vi "ImageBrowser.vi"() -> ()   [LabVIEW 2016]
doc: "This example shows how to set up an image browser. An image browser is a concise representation of the images in your database represented as thumbnails on a page. You can use the Browser VIs in NI Vision to configure a browser, configure the selection of one or many images, add new images and remove images to and from a browser, replace an image, and get or set the selection status of an image."
uses:
  <vilib>/vision/NI_Vision_Development_Module.lvlib
panel:
  out "Images":T1(plugin-control)
  in  "Stop":bool
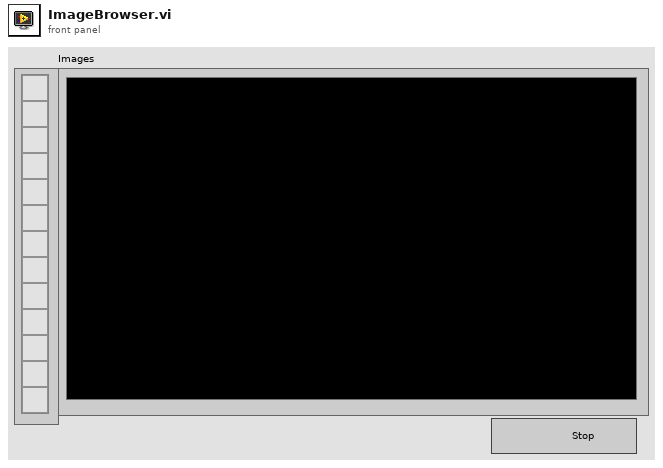
[diagram p1: front panel]
types:
  T1 = typedef "IMAQ Image.ctl" = refnum<image>
  T2 = cluster{"Browser\nSize":cluster{"X":i32, "Y":i32}, "Images per Line":i32, "Background Color":u32, "Frame Size":i32, "Frame Style":u16}
  T3 = typedef "Image Type" = u32
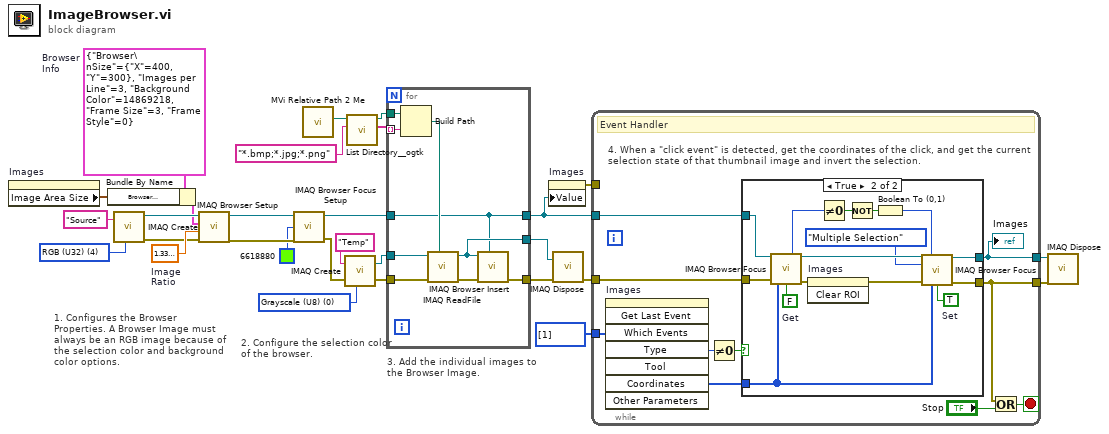
[diagram p0: block diagram]
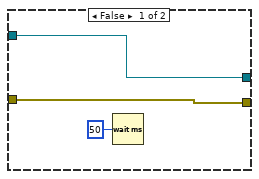
[diagram p2: hidden frame]
diagram:
  w18 = i32[] [1] items=["No Event"=0, "Click Event"=1, "Draw Event"=2, "Size Event"=4, "Scroll Event"=5, "Double Click Event"=8] ("Which Events")
  w29 = sgl 1.33  # Image  Ratio
  w8 = T2 {"Browser\nSize"={"X"=400, "Y"=300}, "Images per Line"=3, "Background Color"=14869218, "Frame Size"=3, "Frame Style"=0}  # Browser Info
  w22 = T3 0 items=["Grayscale (U8)", "Grayscale (I16)", "Grayscale (SGL)", "Complex (CSG)", "RGB (U32)", "HSL (U32)", "RGB (U64)", "Grayscale (U16)"] ("Image Type")
  w24 = T3 4 items=["Grayscale (U8)", "Grayscale (I16)", "Grayscale (SGL)", "Complex (CSG)", "RGB (U32)", "HSL (U32)", "RGB (U64)", "Grayscale (U16)"] ("Image Type")
  # "3. Add the individual images to the Browser Image."
  # "2. Configure the selection color of the browser."
  # "1. Configures the Browser Properties. A Browser Image must always be an RGB image because of the selection color and background color options."
  n1 = property on="Images" class="ImageControl"() -> ("Image Area Size"=w7:cluster{"Width":u32, "Height":u32})  [unwired: 2 in, 2 out]
  n2 = Bundle By Name(cluster=w8, "Browser\nSize"=w7) -> (w6:T2)
  n3 = call "IMAQ Create"("Image Name"="Source", "Image Type"=w24) -> ("New Image"=w26:T1, "error out"=w25:errorcluster)  [unwired: 3 in]
  n4 = call "IMAQ Browser Setup"("error in (no error)"=w25, "Image Ratio"=w29, "Browser Info"=w6, "Image In"=w26) -> ("error out"=w12:errorcluster, "Image Browser Out"=w13:T1)  [unwired: 2 out]
  n5 = call "IMAQ Browser Focus Setup"("error in (no error)"=w12, "Focus Color"=u32 6618880, "Image Browser In"=w13) -> ("error out"=w10:errorcluster, "Image Browser Out"=w11:T1)  [unwired: 1 in]
  n6 = call "MVi Relative Path 2 Me.vi"() -> ("MyDir"=w1:path)  [unwired: 6 in, 1 out]
  n7 = call "IMAQ Create"("Image Name"="Temp", "Image Type"=w22, "error in (no error)"=w10) -> ("New Image"=w15:T1, "error out"=w28:errorcluster)  [unwired: 2 in]
  n8 = call "List Directory__ogtk.vi"("pattern"="*.bmp;*.jpg;*.png", "directory path"=w1) -> ("file names"=w2:string[], "dup directory path"=w4:path)  [unwired: 2 in, 2 out]
  n9 = for {
    tunnel: w11 -> [w30]
    tunnel: w4 -> [w38]
    tunnel: w2 -> [w35] mode=indexing
    tunnel: w28 -> [w34]
    tunnel: [w33] -> w27
    tunnel: [w30] -> w19
    tunnel: w15 -> [w32]
    tunnel: [w31] -> w14
    n10 = Build Path(base path=w38, name or relative path=w35) -> (appended path=w37:path)
    n11 = call "IMAQ ReadFile"("File Path"=w37, "error in (no error)"=w34, "Image"=w32) -> ("error out"=w36:errorcluster, "Image Out"=w31:T1)  [unwired: 4 in, 3 out]
    n12 = call "IMAQ Browser Insert"("Image Browser In"=w30, "error in (no error)"=w36, "Image to Add"=w31) -> ("error out"=w33:errorcluster)  [unwired: 4 in, 4 out]
  }
  n13 = property on="Images" class="ImageControl"("Value"=w19) -> (error out=w5:errorcluster)  [unwired: 2 in, 1 out]
  n14 = call "IMAQ Dispose"("Image"=w14, "error in (no error)"=w27) -> ("error out"=w20:errorcluster)  [unwired: 4 in]
  n15 = while {
    tunnel: w19 -> [w48]
    tunnel: w20 -> [w45]
    tunnel: w18 -> [w46]
    tunnel: [w43] -> w17
    tunnel: [w40] -> w16
    tunnel: w5 -> [_]
    stop <- w41 stop-if-true
    # "4. When a \"click event\" is detected, get the coordinates of the click, and get the current selection state of that thumbnail image and invert the selection."
    # "Event Handler"
    n16 = invoke on="Images" class="ImageControl" method="Get Last Event"("Which Events"=w46) -> ("Type"=w39:i32, "Coordinates"=w47:i32[])  [unwired: 7 in, 6 out]
    n17 = Not Equal To 0?(x=w39) -> (x != 0?=w44:bool)
    n18 = case shown="True" w44 {
      tunnel: w48 -> [w50 w66]
      tunnel: w47 -> [_ w57]
      tunnel: w45 -> [w51 w56]
      tunnel: [w51 w55] -> w43
      tunnel: [w50 w54] -> w40
      frame False {
        n19 = Wait (ms)(milliseconds to wait=u32 50) -> ()  [unwired: 1 out]
      }
      frame True {
        w64 = TRUE  # Set
        w65 = FALSE  # Get
        n20 = call "IMAQ Browser Focus"("Image Browser In"=w66, "error in (no error)"=w56, "Pixel Position"=w57, "Get/Set (Set)"=w65) -> ("State Out"=w61:enum16{"Not selected", "Selected"}, "Image Browser Out"=w63:T1, "error out"=w53:errorcluster)  [unwired: 6 in, 3 out]
        n21 = invoke on="Images" class="ImageControl" method="Clear ROI"(error in=w53) -> (error out=w52:errorcluster)  [unwired: 2 in, 2 out]
        n22 = Not Equal To 0?(x=w61) -> (x != 0?=w59:bool)
        n23 = Not(x=w59) -> (.not. x?=w58:bool)
        n24 = Boolean To (0,1)(Boolean=w58) -> (0, 1=w60:i16)
        n25 = call "IMAQ Browser Focus"("Image Browser In"=w63, "State In"=w60, "Selection Mode"=enum16{"Single Selection", "Multiple Selection"}."Multiple Selection", "error in (no error)"=w52, "Pixel Position"=w57, "Get/Set (Set)"=w64) -> ("Image Browser Out"=w54:T1, "error out"=w55:errorcluster)  [unwired: 4 in, 4 out]
      }
    }
    "Images" <- w40
    n26 = Or(x=w43, y="Stop") -> (x .or. y?=w41:bool)
  }
  n27 = call "IMAQ Dispose"("Image"=w16, "error in (no error)"=w17) -> ()  [unwired: 4 in, 1 out]
